vi "Constructor.vi"(7 "Peeping?":bool, 8 "error in (no error)":errorcluster, 11 "Path":path) -> (0 "error out":errorcluster, 3 "Block Diagram":refnum<class "VI.lvclass">)   [LabVIEW 2026, in "VI.lvclass"]
doc: "Create all the high level structure classes and get all the references to start the scripting."
uses:
  VI.lvclass
  Main Sequence/Main Sequence.lvclass
  DMA Loop/DMA Loop.lvclass
  VI.lvclass/VI.ctl
  Module Loop/Module Loop.lvclass
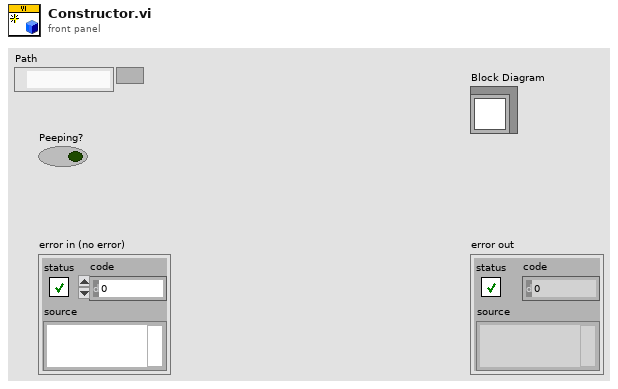
[diagram p1: front panel]
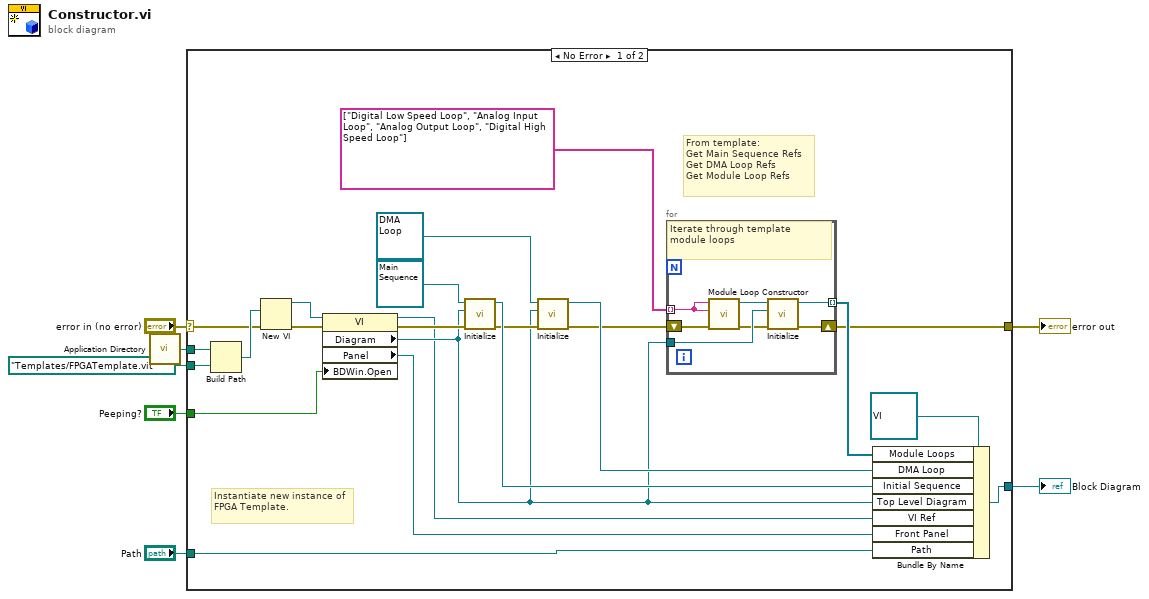
[diagram p0: block diagram]
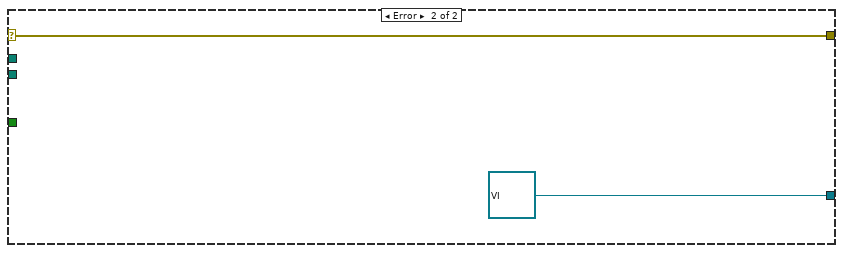
[diagram p2: hidden frame]
diagram:
  n1 = call <vilib>:"Application Directory.vi"() -> ("Application Directory"=w5:path)
  n2 = case shown="No Error" "error in (no error)" {
    selector: "error in (no error)" -> [w14 w39]
    tunnel: [w26 refnum<class "VI.lvclass"> refnum ("Block Diagram.lvclass")] -> w7
    tunnel: [w23 w39] -> w6
    tunnel: w5 -> [w21 _]
    tunnel: path "Templates/FPGATemplate.vit" ("Application Directory") -> [w20 _]
    tunnel: "Path" -> [w11 _]
    tunnel: "Peeping?" -> [w8 _]
    frame No Error {
      # "From template:\nGet Main Sequence Refs\nGet DMA Loop Refs\nGet Module Loop Refs"
      # "Instantiate new instance of FPGA Template."
      n3 = Build Path(base path=w21, name or relative path=w20) -> (appended path=w19:path)
      n4 = New VI(8:w14, 10:w19) -> (0:w17:errorcluster, 3:w18:refnum<vi>)  [unwired: 5 in]
      n5 = property class="VI"(reference=w18, error in=w17, "BDWin.Open"=w8) -> (reference out=w9:refnum<vi>, error out=w16:errorcluster, "Diagram"=w15:refnum<vi>, "Panel"=w10:refnum<vi>)
      n6 = call-dynamic "Initialize.vi"("error in (no error)"=w16, "Top Level Diagram"=w15, "Initial Sequence in"=refnum<class "Main Sequence.lvclass"> refnum ("Initial Sequence.lvclass")) -> ("error out"=w27:errorcluster, "Initial Sequence out"=w28:refnum<class "Main Sequence.lvclass">)  [unwired: 7 in]
      n7 = call-dynamic "Initialize.vi"("error in (no error)"=w27, "Top Level Diagram"=w15, "DMA Loop in"=refnum<class "DMA Loop.lvclass"> refnum ("DMA Loop.lvclass")) -> ("error out"=w24:errorcluster, "DMA Loop out"=w29:refnum<class "DMA Loop.lvclass">)  [unwired: 7 in]
      n8 = for {
        tunnel: w15 -> [w36]
        shift-right: [w37] -> w23
        shift-left: w24 -> [w33]
        tunnel: [w35] -> w25 mode=indexing
        tunnel: string[] ["Digital Low Speed Loop", "Analog Input Loop", "Analog Output Loop", "Digital High Speed Loop"] -> [w31] mode=indexing
        # "Iterate through template module loops"
        n9 = call "Module Loop Constructor.vi"("error in (no error)"=w33, "Name"=w31, "Type"=w31) -> ("error out"=w32:errorcluster, "Module Loop.lvclass"=w34:refnum<class "Module Loop.lvclass">)  [unwired: 7 in]
        n10 = call-dynamic "Initialize.vi"("error in (no error)"=w32, "Top Level Diagram"=w36, "IO Loop in"=w34) -> ("error out"=w37:errorcluster, "IO Loop out"=w35:refnum<class "Module Loop.lvclass">)  [unwired: 7 in]
      }
      n11 = Bundle By Name(cluster=refnum<class "VI.lvclass"> refnum ("Block Diagram.lvclass"), "Module Loops"=w25, "DMA Loop"=w29, "Initial Sequence"=w28, "Top Level Diagram"=w15, "VI Ref"=w9, "Front Panel"=w10, "Path"=w11) -> (w26:refnum<class "VI.lvclass">)
    }
    frame Error {
    }
  }
  "Block Diagram" <- w7
  "error out" <- w6
